vi "Write_Wrap.vi"(8 "error in (no error)":errorcluster, 10 "Value":T1, 11 "Var_DBL in":refnum<class "Var_DBL.lvclass">) -> (0 "error out":errorcluster, 3 "Var_DBL out":refnum<class "Var_DBL.lvclass">)   [LabVIEW 2021, in "Var_DBL.lvclass"]
uses:
  Var_DBL.lvclass
  Type.ctl
  Var_DBL.lvclass/Var_DBL.ctl
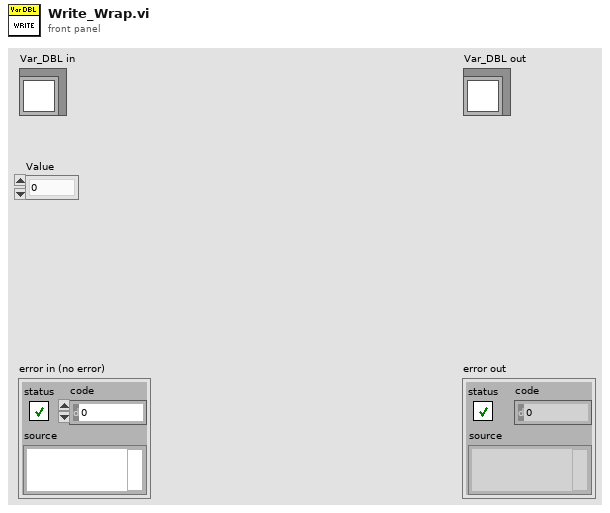
[diagram p1: front panel]
types:
  T1 = typedef "Var_DBL.lvclass/Type.ctl" = dbl
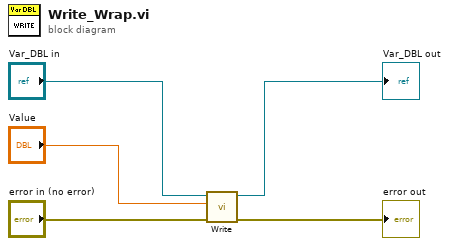
[diagram p0: block diagram]
diagram:
  n1 = call-dynamic "Write.vi"("error in (no error)"="error in (no error)", "Value"="Value", "Double Float.lvclass_340760 in"="Var_DBL in") -> ("error out"=→"error out":errorcluster, "Double Float.lvclass_340760 out"=→"Var_DBL out":refnum<class "Var_DBL.lvclass">)  [unwired: 7 in]
